vi "PhotEyeCount.vi"(7 "Enum":enum16{"Count", "Reset"}(ring)=enum."Reset") -> (2 "count":i32)   [LabVIEW 2023]
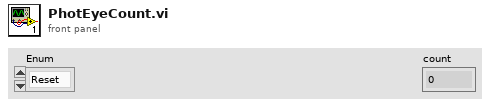
[diagram p1: front panel]
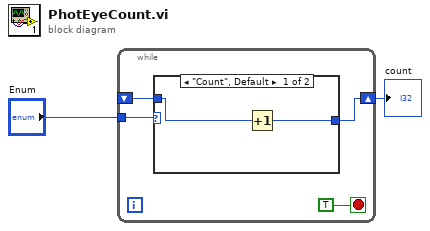
[diagram p0: block diagram]
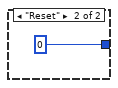
[diagram p2: hidden frame]
diagram:
  n1 = while {
    tunnel: "Enum" -> [w5]
    shift-right: [w4] -> w1
    shift-left: _ -> [w3]
    stop <- TRUE stop-if-true
    n2 = case shown="\"Count\", Default" w5 {
      tunnel: [w7 0] -> w4
      tunnel: w3 -> [w8 _]
      frame "Count", Default {
        n3 = Increment(x=w8) -> (x+1=w7:i32)
      }
      frame "Reset" {
      }
    }
  }
  "count" <- w1
